vi "SaveOneSweep.vi"(5 "Position":T1[](array[typedef]), 7 "SectionProperties":T3, 8 "error in (no error)":errorcluster, 9 ".csv file from N5222A":string, 10 "Temperature, deg C":dbl, 11 "DataLogRaster in":refnum<class "DataLogRaster.lvclass">) -> (0 "error out":errorcluster, 3 "DataLogRaster out":refnum<class "DataLogRaster.lvclass">)   [LabVIEW 2019, in "DataLogRaster.lvclass"]
uses:
  DataLogRaster.lvclass
  Datalog/DatalogSubvis/SearchableTag.ctl
  Sequence/SequenceSubvis/RF Direction.ctl
  Sequence/SequenceSubvis/PolarizationSelect.ctl
  APARMainSubvis/VXM Public API/singleAxisMoveDef.ctl
  APARMainSubvis/VXM Public API/mmWaveAxis.ctl
  DataLogRaster.lvclass/DataLogRaster.ctl
  Datalog/DataLog.lvclass
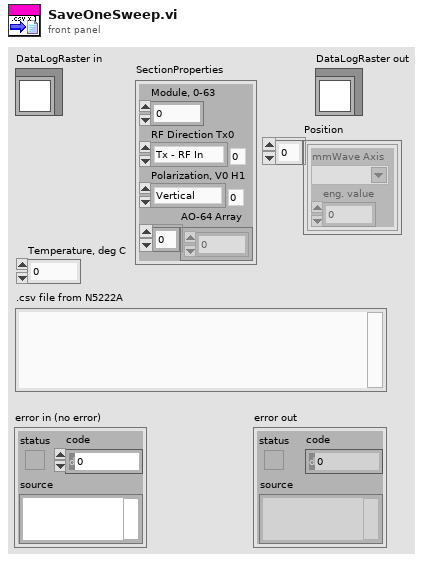
[diagram p1: front panel]
types:
  T1 = typedef "singleAxisMoveDef.ctl" = cluster{"mmWave Axis":T2, "eng. value":dbl}
  T2 = typedef "mmWaveAxis.ctl" = string
  T3 = typedef "DataLog.lvclass/SearchableTag.ctl" = cluster{"Module, 0-63":i32, "RF Direction Tx0":T4, "Polarization, V0 H1":T5, "AO-64 Array":dbl[]}
  T4 = typedef "RF Direction.ctl" = enum16{"Tx - RF In", "Rx - RF Out"}
  T5 = typedef "PolarizationSelect.ctl" = enum16{"Vertical", "Horizontal"}
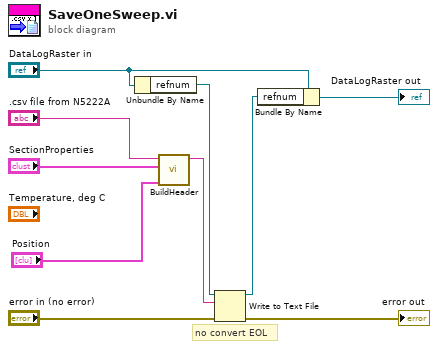
[diagram p0: block diagram]
diagram:
  # "no convert EOL"
  n1 = Unbundle By Name("DataLogRaster in") -> ("refnum"=w5:refnum<file>)
  n2 = call "BuildHeader.vi"("Moves"="Position", "SectionProperties"="SectionProperties", "PNA .csv File"=".csv file from N5222A") -> ("One Record"=w6:string)  [unwired: 8 in]
  n3 = Write to Text File(file (use dialog)=w5, text=w6, error in="error in (no error)") -> (refnum out=w4:refnum<file>, error out=→"error out":errorcluster)  [unwired: 1 in, 1 out]
  n4 = Bundle By Name(cluster="DataLogRaster in", "refnum"=w4) -> (→"DataLogRaster out":refnum<class "DataLogRaster.lvclass">)
